vi "JSON-ActorCommand.vi"(6 "Payload":string="Inventory", 8 "error in":errorcluster, 9 "Reply Command":string="ReplyWithAddQuery", 10 "SQL Statement":string, 11 "Table":string="Inventory") -> (0 "error out":errorcluster, 3 "Output JSON Object":string)   [LabVIEW 2013]
uses:
  ftw-dataflow/Actor/src/Utility/FTW-Actor-Configuration.ctl
  ftw-dataflow/Actor/src/FTW-Actor.lvlib
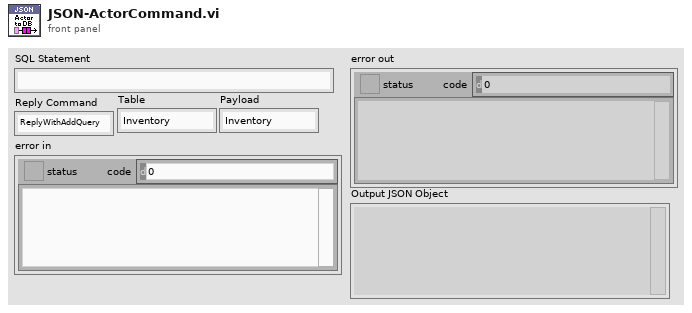
[diagram p1: front panel]
types:
  T1 = typedef "FTW-Actor.lvlib/FTW-Actor-Configuration.ctl" = string
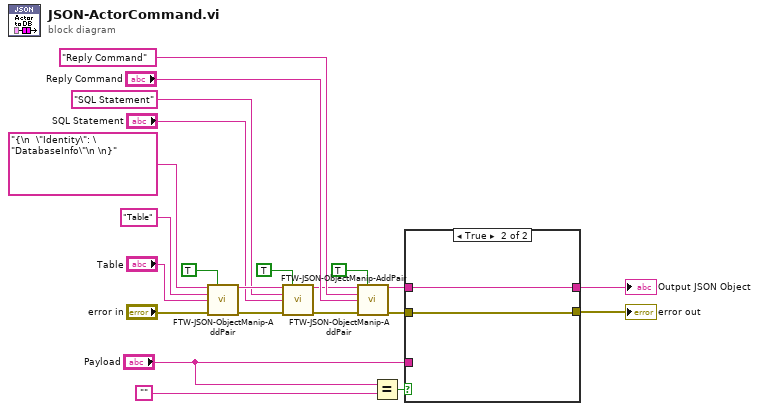
[diagram p0: block diagram]
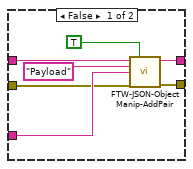
[diagram p2: hidden frame]
diagram:
  n1 = call "FTW-JSON-ObjectManip-AddPair.vi"("Input JSON Object"=T1 "{\n  \"Identity\": \"DatabaseInfo\"\n \n}" ("FTW Actor Instance Configuration 2"), "Escape Value to String?"=TRUE, "Key"="Table", "Value"="Table", "error in"="error in") -> ("Output JSON Object"=w18:string, "error out"=w9:errorcluster)  [unwired: 9 in]
  n2 = call "FTW-JSON-ObjectManip-AddPair.vi"("Input JSON Object"=w18, "Escape Value to String?"=TRUE, "Key"="SQL Statement", "Value"="SQL Statement", "error in"=w9) -> ("Output JSON Object"=w20:string, "error out"=w8:errorcluster)  [unwired: 9 in]
  n3 = call "FTW-JSON-ObjectManip-AddPair.vi"("Input JSON Object"=w20, "Escape Value to String?"=TRUE, "Key"="Reply Command", "Value"="Reply Command", "error in"=w8) -> ("Output JSON Object"=w7:string, "error out"=w3:errorcluster)  [unwired: 9 in]
  n4 = Equal?(x="Payload", y="") -> (x = y?=w6:bool)
  n5 = case shown="True" w6 {
    tunnel: w7 -> [w28 w31]
    tunnel: "Payload" -> [w26 _]
    tunnel: w3 -> [w25 w30]
    tunnel: [w24 w30] -> w2
    tunnel: [w23 w31] -> w1
    frame False {
      n6 = call "FTW-JSON-ObjectManip-AddPair.vi"("Input JSON Object"=w28, "Escape Value to String?"=TRUE, "Key"="Payload", "Value"=w26, "error in"=w25) -> ("Output JSON Object"=w23:string, "error out"=w24:errorcluster)  [unwired: 9 in]
    }
    frame True {
    }
  }
  "error out" <- w2
  "Output JSON Object" <- w1
